vi "Hipot_Init.vi"(8 "Error In":errorcluster, 10 "PORT":string, 11 "Limit":string="1240~5~1~1") -> (0 "error out":errorcluster, 2 "Result":bool, 3 "Data":string)   [LabVIEW 2013]
panel:
  out "Error Out":errorcluster
  out "CMD":string[](array[string])
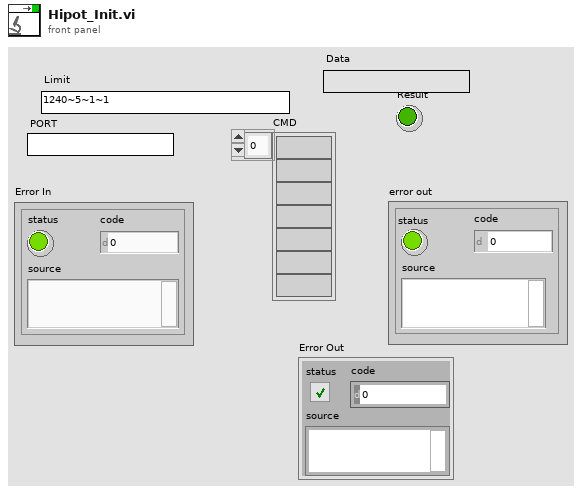
[diagram p1: front panel]
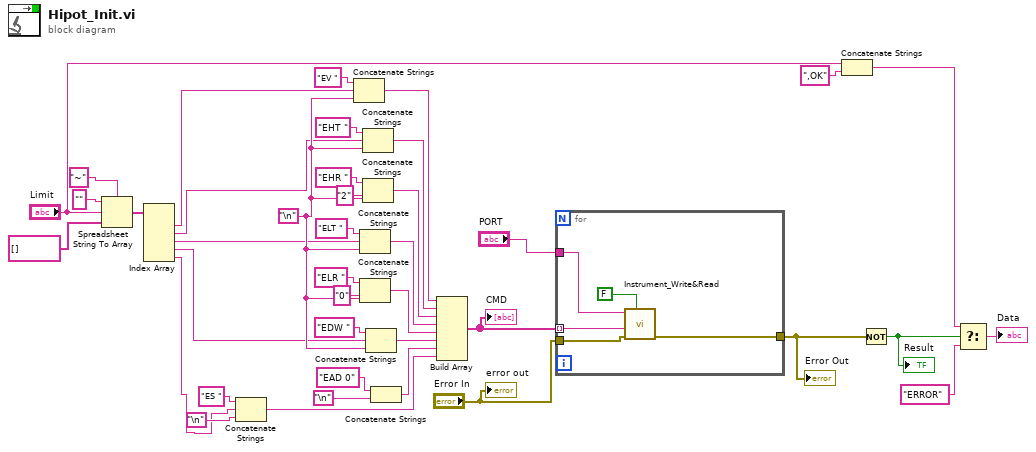
[diagram p0: block diagram]
diagram:
  w15 = "\n"
  n1 = Spreadsheet String To Array(delimiter (Tab)="~", format string="", spreadsheet string="Limit", array type (2D Dbl)=string[] []) -> (array=w25:string[])
  n2 = Index Array(array=w25) -> (element #1=w24:string, element #2=w11:string, element #3=w10:string, element #4=w3:string, element #5=w2:string)  [unwired: 5 in]
  n3 = Concatenate Strings("ES " ("写入缓冲区"), w2, "\n") -> (w17:string)
  n4 = Concatenate Strings("EV " ("字符串"), w24, w15) -> (w30:string)
  n5 = Concatenate Strings("ELT " ("字符串"), w10, w15) -> (w9:string)
  n6 = Concatenate Strings("ELR " ("字符串"), "0" ("string"), w15) -> (w8:string)
  n7 = Concatenate Strings("EHT " ("字符串"), w11, w15) -> (w29:string)
  n8 = Concatenate Strings("EHR " ("字符串"), "2" ("string"), w15) -> (w28:string)
  n9 = Concatenate Strings("EDW " ("字符串"), w3, w15) -> (w7:string)
  n10 = Concatenate Strings("EAD 0" ("写入缓冲区"), "\n") -> (w6:string)
  n11 = Build Array(w30, w29, w28, w9, w8, w7, w6, w17) -> (w27:string[])
  "CMD" <- w27
  n12 = for {
    tunnel: "PORT" -> [w44]
    tunnel: "Error In" -> [w41]
    tunnel: w27 -> [w45] mode=indexing
    tunnel: [w42] -> w40
    n13 = call "Instrument_Write&Read.vi"("Read?"=FALSE, "Error In"=w41, "CMD"=w45, "PORT"=w44) -> ("Error Out"=w42:errorcluster)  [unwired: 6 in, 1 out]
  }
  "Error Out" <- w40
  n14 = Concatenate Strings("Limit", ",OK") -> (w19:string)
  n15 = Not(x=w40) -> (.not. x?=w37:bool)
  "Result" <- w37
  n16 = Select(t=w19, s=w37, f="ERROR") -> (s? t:f=→"Data":string)
  "error out" <- "Error In"
